vi "Get Sensitivity.vi"() -> (3 "Sensitivity":dbl)   [LabVIEW 2014]
uses:
  <vilib>/Rock Robotics/Network Tables/SD Read Number.vi
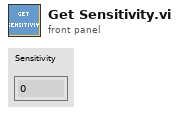
[diagram p1: front panel]
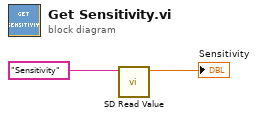
[diagram p0: block diagram]
diagram:
  n1 = call-poly <vilib>:"SD Read Value.vi"("Name"="Sensitivity") -> ("Numeric"=→"Sensitivity":dbl)  [unwired: 8 in, 2 out]
